vi "CaseStructure1.vi"() -> ()   [LabVIEW 2015]
panel:
  out "Boolean":bool
  in  "OK Button 4":bool
  in  "OK Button 3":bool
  in  "OK Button 2":bool
  in  "OK Button":bool
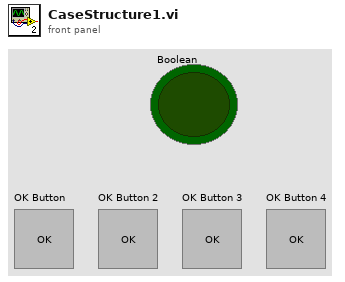
[diagram p1: front panel]
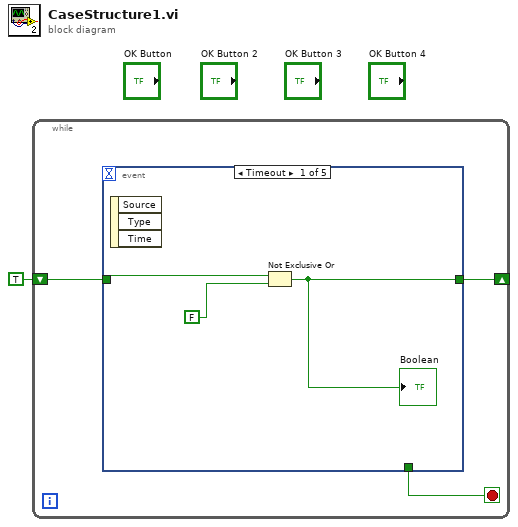
[diagram p0: block diagram]
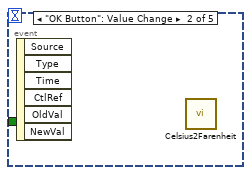
[diagram p2: hidden frame]
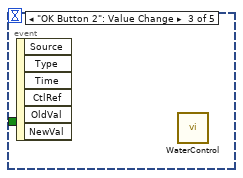
[diagram p3: hidden frame]
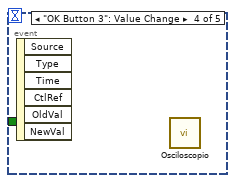
[diagram p4: hidden frame]
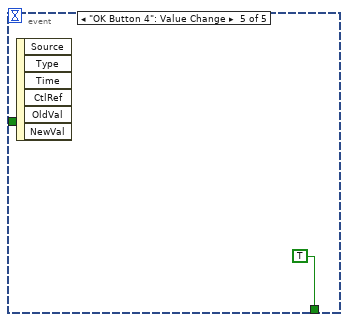
[diagram p5: hidden frame]
diagram:
  n1 = while {
    shift-right: [w4] -> _
    shift-left: TRUE -> [w3]
    stop <- w2 stop-if-true
    n2 = event shown="[0] Timeout" {
      selector: _ -> [_ _ _ _ _]
      dyn-events: _ -> [_ _ _ _ _]
      timeout: _ -> [_ _ _ _ _]
      tunnel: [w6 _ _ _ _] -> w4
      tunnel: w3 -> [w5 _ _ _ _]
      tunnel: [_ _ _ _ TRUE] -> w2
      event Timeout {
        n3 = event-data() -> ()  [unwired: 1 in, 3 out]
        n4 = Not Exclusive Or(1:FALSE, 2:w5) -> (0:w6:bool)
        "Boolean" <- w6
      }
      event "OK Button": Value Change {
        n5 = event-data() -> ()  [unwired: 1 in, 6 out]
        n6 = call "Celsius2Farenheit.vi"() -> ()  [unwired: 1 in, 2 out]
      }
      event "OK Button 2": Value Change {
        n7 = event-data() -> ()  [unwired: 1 in, 6 out]
        n8 = call "WaterControl.vi"() -> ()  [unwired: 12 in]
      }
      event "OK Button 3": Value Change {
        n9 = event-data() -> ()  [unwired: 1 in, 6 out]
        n10 = call "Osciloscopio.vi"() -> ()  [unwired: 12 in]
      }
      event "OK Button 4": Value Change {
        n11 = event-data() -> ()  [unwired: 1 in, 6 out]
      }
    }
  }
